vi "Destroy.vi"(8 "error in (no error)":errorcluster, 11 "Plugin Manager in":refnum<class "CIFPluginLoader.lvclass">) -> (0 "error out":errorcluster, 3 "Plugin Manager out":refnum<class "CIFPluginLoader.lvclass">)   [LabVIEW 2021, in "CIFPluginLoader.lvclass"]
uses:
  CIFPluginLoader.lvclass
  <vilib>/CIF Foundation/CIF Core/CIFPluginManager/gRPC/CIF_Manager_client/RPC Messages/cif_manager_UnregisterPluginLoaderRequest.ctl
  <vilib>/CIF Foundation/CIF Core/CIFUtilities/CIFLogs/Typedef/Message Type.ctl
  CIFPluginLoader.lvclass/CIFPluginLoader.ctl
  <vilib>/CIF Foundation/CIF Core/CIFUtilities/CIFLogs/CIFLogs.lvlib
  <vilib>/CIF Foundation/CIF Core/CIFPluginManager/gRPC/CIF_Manager_Client_Wrapper/CIFManagerClientWrapper.lvlib
  <vilib>/CIF Foundation/CIF Core/CIFUtilities/CIFConfigurationFile/CIF Configuration File.lvlib
  <vilib>/CIF Foundation/CIF Core/CIFPluginManager/gRPC/CIF_Manager_client/CIF_Manager_client.lvlib
  gRPC/CIF_PluginLoader_server/RPC Service/PluginLoader/PluginLoader.lvclass
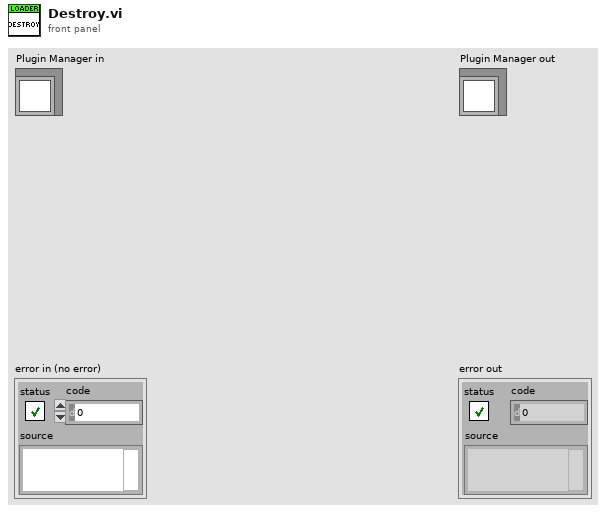
[diagram p1: front panel]
types:
  T1 = typedef "CIF_Manager_client.lvlib/cif_manager_UnregisterPluginLoaderRequest.ctl" = cluster{"loader_name":string}
  T2 = typedef "CIFLogs.lvlib/Message Type.ctl" = enum8{"Error", "Information", "Print Terminal", "Configuration"}
  T3 = typedef "grpc-lvsupport-release.lvlib/grpcId.ctl" = u64
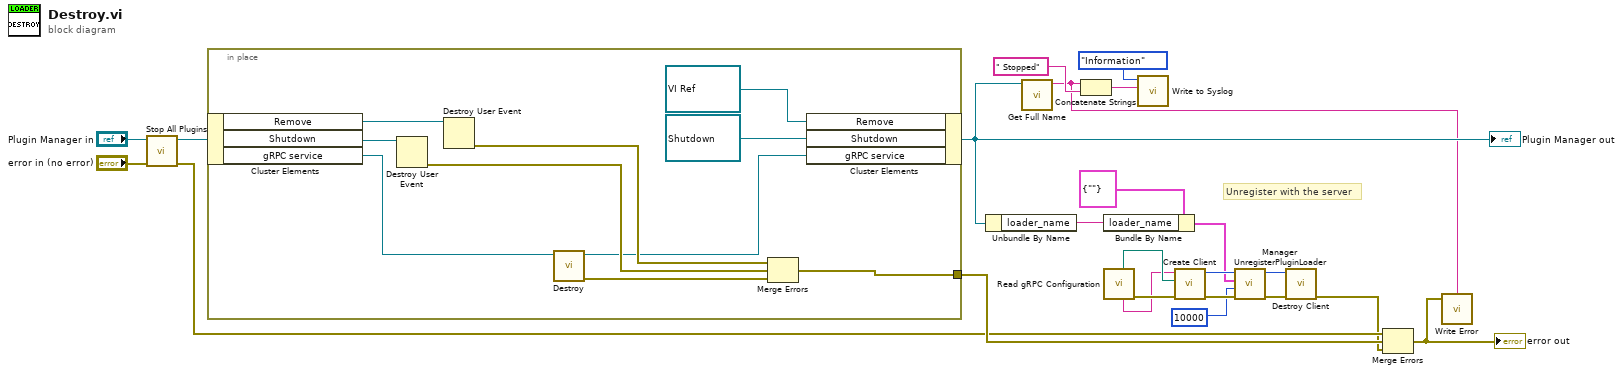
[diagram p0: block diagram]
diagram:
  # "Unregister with the server"
  n1 = call "Stop All Plugins.vi"("error in (no error)"="error in (no error)", "CIFPluginLoader in"="Plugin Manager in") -> ("error out"=w16:errorcluster, "CIFPluginLoader out"=w18:refnum<class "CIFPluginLoader.lvclass">)  [unwired: 8 in]
  n2 = in-place {
    in-place-border: [w32] -> w23
    n3 = in-place-cluster #1(w18) -> ("Remove"=w28:refnum<user-event>, "Shutdown"=w31:refnum<user-event>, "gRPC service"=w25:refnum<class "PluginLoader.lvclass">)
    n4 = Destroy User Event(user event=w31) -> (error out=w30:errorcluster)  [unwired: 1 in]
    n5 = Destroy User Event(user event=w28) -> (error out=w27:errorcluster)  [unwired: 1 in]
    n6 = call-dynamic "Destroy.vi"("gRPC service in"=w25) -> ("error out"=w33:errorcluster, "gRPC service out"=w24:refnum<class "PluginLoader.lvclass">)  [unwired: 9 in]
    n7 = Merge Errors(w27, w30, w33) -> (w32:errorcluster)
    n8 = in-place-cluster #1("Remove"=refnum<user-event> refnum ("Parallel Events.Remove"), "Shutdown"=refnum<user-event> refnum ("Parallel Events.Shutdown"), "gRPC service"=w24) -> (w6:refnum<class "CIFPluginLoader.lvclass">)
  }
  "Plugin Manager out" <- w6
  n9 = Unbundle By Name(w6) -> ("loader_name"=w5:string)
  n10 = call "Get Full Name.vi"("CIFPluginLoader in"=w6) -> ("Name"=w1:string)  [unwired: 10 in]
  n11 = Concatenate Strings(w1, " Stopped" ("message")) -> (w20:string)
  n12 = Bundle By Name(cluster=T1 {"loader_name"=""} ("Request Data"), "loader_name"=w5) -> (w4:T1)
  n13 = call <vilib>:"Read gRPC Configuration.vi"() -> ("error out"=w11:errorcluster, "Local Manager Address"=w9:string, "Server Key File (.key)"=w10:path)  [unwired: 6 in, 3 out]
  n14 = call <vilib>:"Write to Syslog.vi"("message"=w20, "CIF Message Type"=Message_Type."Information") -> ()  [unwired: 9 in, 1 out]
  n15 = call <vilib>:"Create Client.vi"("error in"=w11, "Server Certificate File (.crt)"=w10, "address"=w9) -> ("error out"=w14:errorcluster, "gRPC ID Out"=w15:T3)  [unwired: 7 in]
  n16 = call <vilib>:"Manager UnregisterPluginLoader.vi"("error in"=w14, "timeout (ms)"=10000, "Request Data"=w4, "gRPC ID"=w15) -> ("error out"=w13:errorcluster, "gRPC ID out"=w12:T3)  [unwired: 5 in, 1 out]
  n17 = call <vilib>:"Destroy Client.vi"("error in"=w13, "gRPC ID"=w12) -> ("error out"=w3:errorcluster)  [unwired: 9 in]
  n18 = Merge Errors(w16, w23, w3) -> (w2:errorcluster)
  "error out" <- w2
  n19 = call <vilib>:"Write Error.vi"("error in (no error)"=w2, "Plugin Name"=w1) -> ()  [unwired: 2 in, 1 out]
